vi "Process SCON_SPOS.vi"(11 "FHPP in":refnum<class "FHPP.lvclass">) -> (3 "FHPP out":refnum<class "FHPP.lvclass">)   [LabVIEW 2022 SP3, in "FHPP.lvclass"]
uses:
  FHPP.lvclass
  FHPP.lvclass/FHPP.ctl
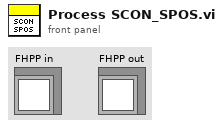
[diagram p1: front panel]
types:
  T1 = typedef "FHPP.lvclass/SPOS.ctl" = cluster{"Halt":bool, "Ack Start":bool, "Motion Complete":bool, "Ack Teach":bool, "Axis Moving":bool, "Drag Error":bool, "Standstill Control":bool, "Axis Referenced":bool}
  T2 = typedef "FHPP.lvclass/SCON.ctl" = cluster{"Drive Enabled":bool, "Operation Enabled":bool, "Warning":bool, "Error":bool, "Load Voltage Applied":bool, "FCT/MMI":bool, "Operation Mode":enum16{"Record Selection", "Direct Mode", "Reserved 1", "Reserved 2"}}
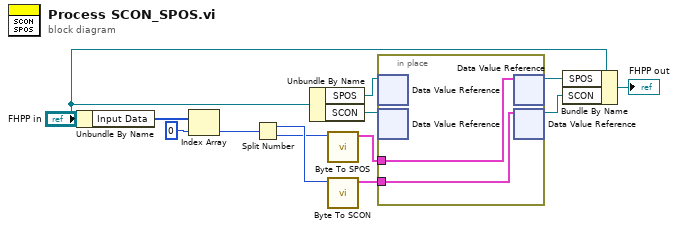
[diagram p0: block diagram]
diagram:
  n1 = Unbundle By Name("FHPP in") -> ("Input Data"=w5:u16[])
  n2 = Index Array(array=w5, index=0) -> (element=w2:u16)
  n3 = Split Number(x=w2) -> (hi(x)=w4:u8, lo(x)=w3:u8)
  n4 = Unbundle By Name("FHPP in") -> ("SPOS"=w7:refnum<data-value>, "SCON"=w8:refnum<data-value>)
  n5 = call "Byte To SPOS.vi"("Numeric"=w3) -> ("SPOS"=w10:T1)  [unwired: 10 in]
  n6 = call "Byte To SCON.vi"("Numeric"=w4) -> ("SCON"=w9:T2)  [unwired: 10 in]
  n7 = in-place {
    in-place-border: w9 -> [w15]
    in-place-border: w10 -> [w14]
    n8 = in-place-dvr #1(w7) -> ()  [unwired: 2 out]
    n9 = in-place-dvr #2(w8) -> ()  [unwired: 2 out]
    n10 = in-place-dvr #1(w14) -> (w12:refnum<data-value>)  [unwired: 1 out]
    n11 = in-place-dvr #2(w15) -> (w13:refnum<data-value>)  [unwired: 1 out]
  }
  n12 = Bundle By Name(cluster="FHPP in", "SPOS"=w12, "SCON"=w13) -> (→"FHPP out":refnum<class "FHPP.lvclass">)
